vi "GetType.vi"(8 "error in (no error)":errorcluster, 11 "Configure Standard Waveform [STD] Msg":refnum<class "Configure Standard Waveform [STD] Msg.lvclass">) -> (0 "error out":errorcluster, 2 "Data Sample":variant, 3 "Configure Standard Waveform [STD] Msg":refnum<class "Configure Standard Waveform [STD] Msg.lvclass">)   [LabVIEW 2015, in "CS++Fgen.lvlib" / "Configure Standard Waveform [STD] Msg.lvclass"]
doc: "This VI delivers a sample of the data type format the message expects."
uses:
  Configure Standard Waveform [STD] Msg.lvclass
  Configure Standard Waveform [STD] Msg.lvclass/Configure Standard Waveform [STD] Msg.ctl
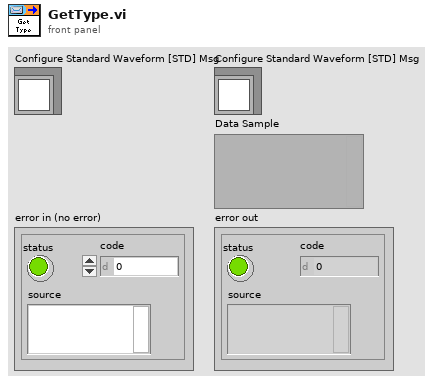
[diagram p1: front panel]
types:
  T1 = cluster{"channel name (\"CHANNEL1\")":string, "waveform (Sine)":i32, "frequency (1000.0 Hz)":dbl[unit], "start phase (0.00 Degrees)":dbl[unit], "amplitude (1.00 V)":dbl[unit], "dc offset (0.00 V)":dbl[unit]}
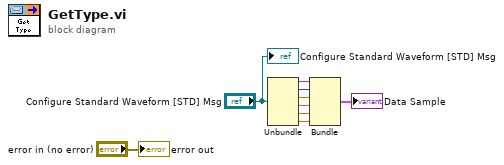
[diagram p0: block diagram]
diagram:
  n1 = Unbundle("Configure Standard Waveform [STD] Msg") -> (w6:string, w5:i32, w4:dbl[unit], w3:dbl[unit], w2:dbl[unit], w1:dbl[unit])
  n2 = Bundle("channel name (\"CHANNEL1\")"=w6, "waveform (Sine)"=w5, "frequency (1000.0 Hz)"=w4, "start phase (0.00 Degrees)"=w3, "amplitude (1.00 V)"=w2, "dc offset (0.00 V)"=w1) -> (→"Data Sample":T1)  [unwired: 1 in]
  "error out" <- "error in (no error)"
  "Configure Standard Waveform [STD] Msg" <- "Configure Standard Waveform [STD] Msg"
